vi "receive.vi"() -> ()   [LabVIEW 2011]
uses:
  RabbitMQ.Client
panel:
  out "string":string
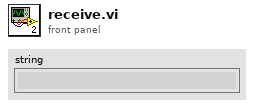
[diagram p1: front panel]
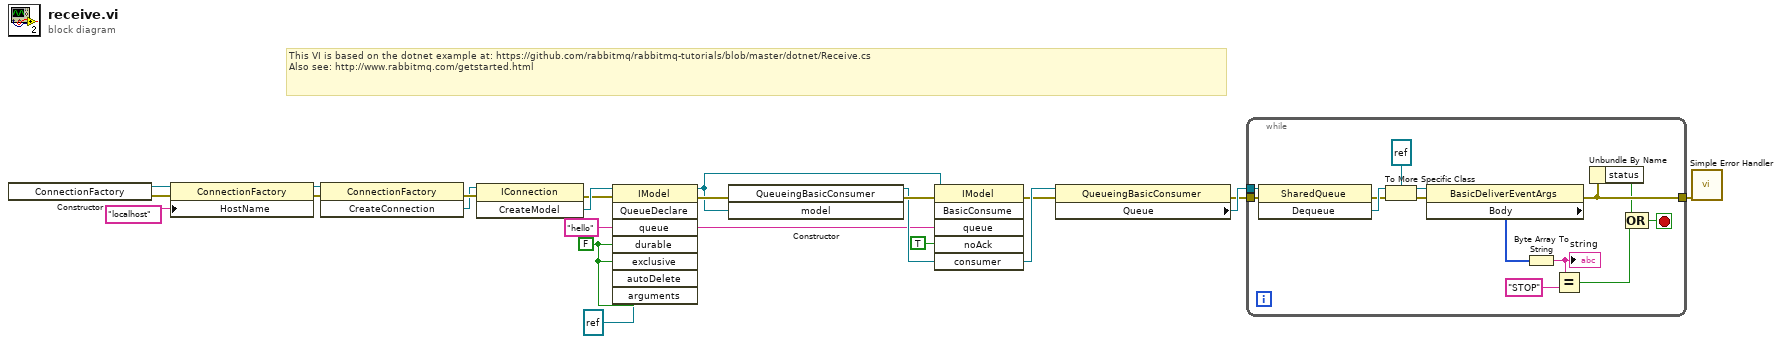
[diagram p0: block diagram]
diagram:
  w12 = FALSE ("durable")
  w4 = "hello" ("queue")
  # "This VI is based on the dotnet example at: https://github.com/rabbitmq/rabbitmq-tutorials/blob/master/dotnet/Receive.cs\nAlso see: http://www.rabbitmq.com/getstarted.html"
  n1 = constructor class="ConnectionFactory"() -> (reference out=w21:refnum<k24>, error out=w19:errorcluster)  [unwired: 3 in, 1 out]
  n2 = property class="ConnectionFactory"(reference=w21, error in=w19, "HostName"="localhost") -> (reference out=w18:refnum<k24>, error out=w17:errorcluster)
  n3 = invoke class="ConnectionFactory" method="CreateConnection"(reference=w18, error in=w17) -> (error out=w16:errorcluster, "CreateConnection"=w15:refnum<k24>)  [unwired: 1 in, 1 out]
  n4 = invoke class="IConnection" method="CreateModel"(reference=w15, error in=w16) -> (error out=w13:errorcluster, "CreateModel"=w14:refnum<k24>)  [unwired: 1 in, 1 out]
  n5 = invoke class="IModel" method="QueueDeclare"(reference=w14, error in=w13, "queue"=w4, "durable"=w12, "exclusive"=w12, "autoDelete"=w12, "arguments"=refnum<k24> refnum) -> (reference out=w1:refnum<k24>, error out=w10:errorcluster)  [unwired: 1 in, 6 out]
  n6 = constructor class="QueueingBasicConsumer"(error in=w10, "model"=w1) -> (reference out=w7:refnum<k24>, error out=w8:errorcluster)  [unwired: 2 in, 2 out]
  n7 = invoke class="IModel" method="BasicConsume"(reference=w1, error in=w8, "queue"=w4, "noAck"=TRUE, "consumer"=w7) -> (error out=w5:errorcluster)  [unwired: 1 in, 5 out]
  n8 = property class="QueueingBasicConsumer"(reference=w7, error in=w5) -> (error out=w2:errorcluster, "Queue"=w3:refnum<k24>)  [unwired: 1 out]
  n9 = while {
    tunnel: [w35] -> w9
    tunnel: w3 -> [w34]
    tunnel: w2 -> [w33]
    stop <- w22 stop-if-true
    n10 = invoke class="SharedQueue" method="Dequeue"(reference=w34, error in=w33) -> (error out=w30:errorcluster, "Dequeue"=w32:refnum<k24>)  [unwired: 1 in, 1 out]
    n11 = To More Specific Class(target class=refnum<k24> refnum ("Dequeue"), reference=w32, error in=w30) -> (specific class reference=w31:refnum<k24>, error out=w29:errorcluster)
    n12 = property class="BasicDeliverEventArgs"(reference=w31, error in=w29) -> (error out=w35:errorcluster, "Body"=w27:u8[])  [unwired: 1 out]
    n13 = Byte Array To String(unsigned byte array=w27) -> (string=w25:string)
    "string" <- w25
    n14 = Equal?(x=w25, y="STOP") -> (x = y?=w23:bool)
    n15 = Unbundle By Name(w35) -> ("status"=w26:bool)
    n16 = Compound Arithmetic op=OR(w26, w23) -> (w22:bool)
  }
  n17 = call <vilib>:"Simple Error Handler.vi"("error in (no error)"=w9) -> ()  [unwired: 4 in, 5 out]
